vi "size saving.vi"(0 "size":dbl[](array[numeric]), 1 "Time for saving":bool, 5 "cSUM":dbl[](array[numeric]), 7 "base path":path, 9 "filename":string="size  ", 11 "error in (no error)":errorcluster, 12 "time  relevant or not?":bool) -> (4 "save done?":bool, 6 "Filename Out":path, 15 "error out":errorcluster)   [LabVIEW 2019]
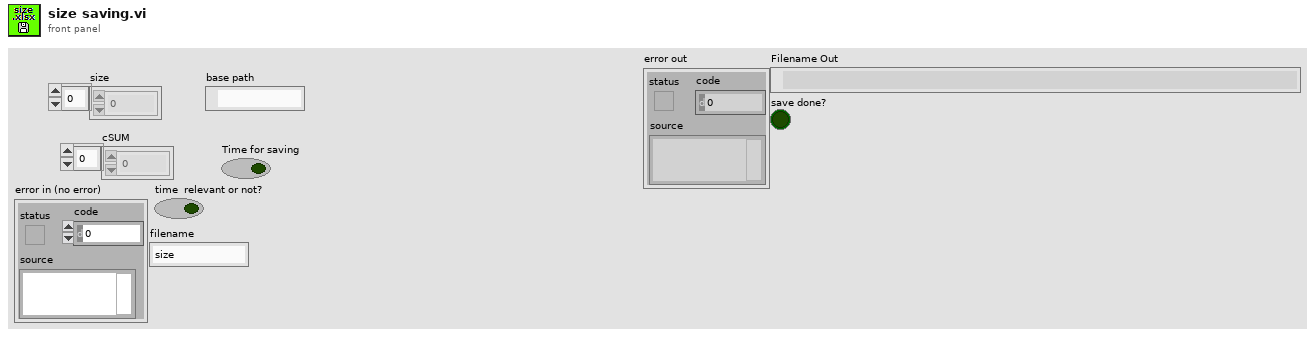
[diagram p1: front panel]
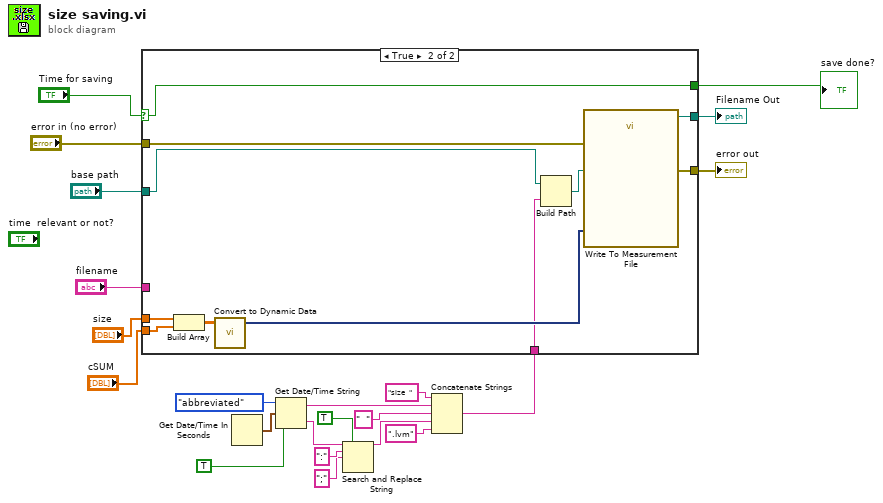
[diagram p0: block diagram]
diagram:
  n1 = Get Date/Time In Seconds() -> (seconds since 1Jan1904=w10:timestamp)
  n2 = Get Date/Time String(date format (0)=enum16{"short", "long", "abbreviated"}."abbreviated", seconds (now)=w10, want seconds? (F)=TRUE) -> (date string=w11:string, time string=w12:string)
  n3 = Search and Replace String(replace all?=TRUE ("replace all? (F)"), input string=w12, search string=":", replace string=";" ("replace string (\"\")")) -> (result string=w13:string)  [unwired: 4 in, 3 out]
  n4 = Concatenate Strings("size  " ("string"), w11, "  " ("string"), w13, ".lvm" ("string")) -> (w2:string)
  n5 = case shown="True" "Time for saving" {
    selector: "Time for saving" -> [w23 w26]
    tunnel: "size" -> [_ w32]
    tunnel: "cSUM" -> [_ w31]
    tunnel: "base path" -> [_ w30]
    tunnel: "error in (no error)" -> [w24 w29]
    tunnel: [w24 w28] -> w17
    tunnel: "filename" -> [_ _]
    tunnel: [_ w27] -> w15
    tunnel: [w23 w26] -> w14
    tunnel: w2 -> [_ w25]
    frame False {
    }
    frame True {
      n6 = Build Array(w32, w31) -> (w34:dbl[][])
      n7 = call "Convert to Dynamic Data"("2D Array"=w34) -> ("Dynamic Data Type"=w33:dynamicdata)  [unwired: 3 in]
      n8 = Build Path(base path=w30, name or relative path=w25) -> (appended path=w35:path)
      n9 = call "Write To Measurement File"("Signals"=w33, "error in (no error)"=w29, "Filename"=w35) -> ("Filename Out"=w27:path, "error out"=w28:errorcluster)  [unwired: 14 in, 1 out]
    }
  }
  "error out" <- w17
  "Filename Out" <- w15
  "save done?" <- w14
